vi "Get JSONEditor Events.vi"(8 "Error In":errorcluster, 11 "WebView.JSONEditor in":refnum<class "WebView.JSONEditor.lvclass">) -> (0 "Error Out":errorcluster, 2 "Events":T1, 3 "WebView.JSONEditor out":refnum<class "WebView.JSONEditor.lvclass">)   [LabVIEW 2020, in "WebView.JSONEditor.lvclass"]
uses:
  WebView.JSONEditor.lvclass
  private/JSONEditor Events.ctl
  private/JSON Updated Event Data--cluster.ctl
  private/Seleced Node Path Event Data--string.ctl
  WebView.JSONEditor.lvclass/WebView.JSONEditor.ctl
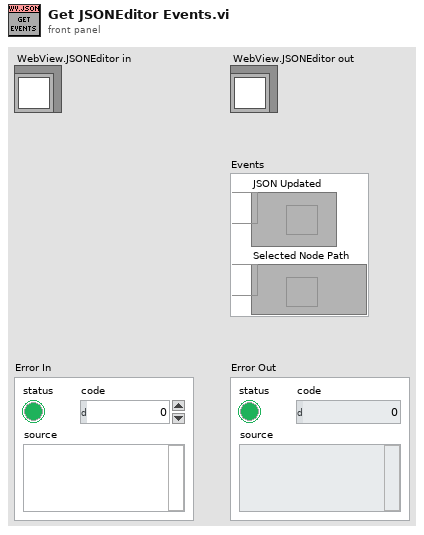
[diagram p1: front panel]
types:
  T1 = typedef "WebView.JSONEditor.lvclass/JSONEditor Events.ctl" = cluster{"JSON Updated":refnum<user-event>, "Selected Node Path":refnum<user-event>}
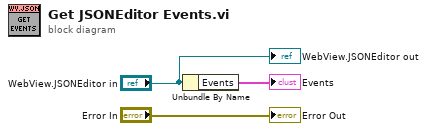
[diagram p0: block diagram]
diagram:
  n1 = Unbundle By Name("WebView.JSONEditor in") -> ("Events"=→"Events":T1)
  "Error Out" <- "Error In"
  "WebView.JSONEditor out" <- "WebView.JSONEditor in"
